vi "PC parse navigation string.vi"(2 "Header":string="T", 3 "Nav String":string="$,A,43,13,230,B,10,20,120,C,10,10,330,D,14,36,110,T,08,12,234\r") -> (0 "Valid?":bool, 1 "Nav Data":T1)   [LabVIEW 2012]
doc: "This VI will parse the Tug navigation string for the Tug letters, A for example, and the time, T. It returns a cluster with the Tug / Time and three values as decimals."
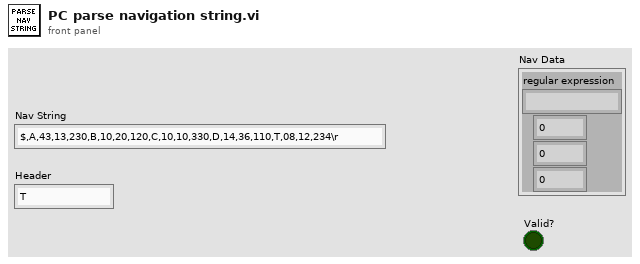
[diagram p1: front panel]
types:
  T1 = cluster{"regular expression":string, i32, i32, i32}
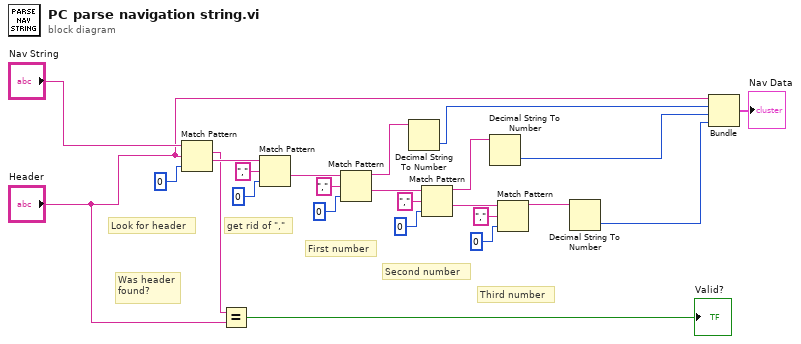
[diagram p0: block diagram]
diagram:
  # "Was header\nfound?"
  # "Third number"
  # "Second number"
  # "First number"
  # "get rid of \",\""
  # "Look for header"
  n1 = Match Pattern(string="Nav String", regular expression="Header", offset (0)=0) -> (match substring=w4:string, after substring=w9:string)  [unwired: 2 out]
  n2 = Equal?(x=w4, y="Header") -> (x = y?=→"Valid?":bool)
  n3 = Match Pattern(string=w9, regular expression=",", offset (0)=0) -> (after substring=w10:string)  [unwired: 3 out]
  n4 = Match Pattern(string=w10, regular expression=",", offset (0)=0) -> (before substring=w21:string, after substring=w17:string)  [unwired: 2 out]
  n5 = Decimal String To Number(string=w21) -> (number=w8:i32)  [unwired: 2 in, 1 out]
  n6 = Match Pattern(string=w17, regular expression=",", offset (0)=0) -> (before substring=w18:string, after substring=w13:string)  [unwired: 2 out]
  n7 = Decimal String To Number(string=w18) -> (number=w1:i32)  [unwired: 2 in, 1 out]
  n8 = Match Pattern(string=w13, regular expression=",", offset (0)=0) -> (before substring=w14:string)  [unwired: 3 out]
  n9 = Decimal String To Number(string=w14) -> (number=w7:i32)  [unwired: 2 in, 1 out]
  n10 = Bundle("Header"="Header", w8, w1, w7) -> (→"Nav Data":cluster{"Header":string, i32, i32, i32})  [unwired: 1 in]
